vi "Network Globals.vi"() -> ()   [LabVIEW 2021]
panel:
  in  "Stop RT":bool
  out "Connected?":bool
  in  "reader endpoint":refnum<k21>
  in  "writer endpoint":refnum<k21>
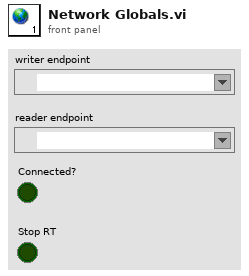
[diagram p1: front panel]
diagram:
